vi "Save Waveform Chart history - single plot.vi"(8 "error in (no error)":errorcluster, 9 "History Data - singple plot":waveform(dbl)[](array[waveform]), 10 "Plot GUI label":string, 11 "Father of all uServices in":refnum<class "Father of all uServices.lvclass">) -> (0 "error out":errorcluster, 3 "Father of all uServices out":refnum<class "Father of all uServices.lvclass">)   [LabVIEW 2026, in "TALOS.lvlib" / "Father of all uServices.lvlib" / "Father of all uServices.lvclass"]
uses:
  Father of all uServices.lvclass
  Waveform Chart Class Reference Strict - single plot.ctl
  Ancestor/Ancestor/Ancestor.lvclass/Ancestor.ctl
  Support VIs/Generate Error.vi
  FGV/Error Memory/Get Error Description.vi
  Support VIs/Get PC name.vi
  Ancestor/Ancestor/Read ID.vi
  Support VIs/Get Class Name.vi
  <vilib>/Utility/error.llb/Clear Errors.vi
  FGV/Error Memory/Error Memory Core.vi
  <vilib>/AdvancedString/Delimited String to 1D String Array.vi
  <vilib>/AdvancedString/Delimited String to 1D String Array (string).vi
  Support VIs/Circus Root Path.vi
  FGV/Error Memory/Error Crt Lvl checker.vi
  FGV/Error Memory/Error Memory Core.vi/40c8088d-b597-4017-91af-faa98e00292e.vi
  FGV/Error Memory/Error Memory Core.vi/d4a3ab98-063c-4e44-b43d-fbdcfe6c2be2.vi
  <vilib>/Utility/file.llb/Write Delimited Spreadsheet (DBL).vi
  Support VIs/Global Memory.vi
  <vilib>/Utility/LVClass/Get LV Class Name.vi
  Support VIs/Is in Packed Library.vi
  Support VIs/TALOS Root path.vi
  Support VIs/Read CSV worksheet.vi
  Support VIs/Global Constants.vi
  <vilib>/Utility/error.llb/General Error Handler.vi
  Support VIs/Error Log.vi
  Ancestor/Ancestor/Ancestor.lvclass
  <vilib>/Comparison/Equal/Equal Functor/Equal Functor.lvclass
  TALOS.lvlib
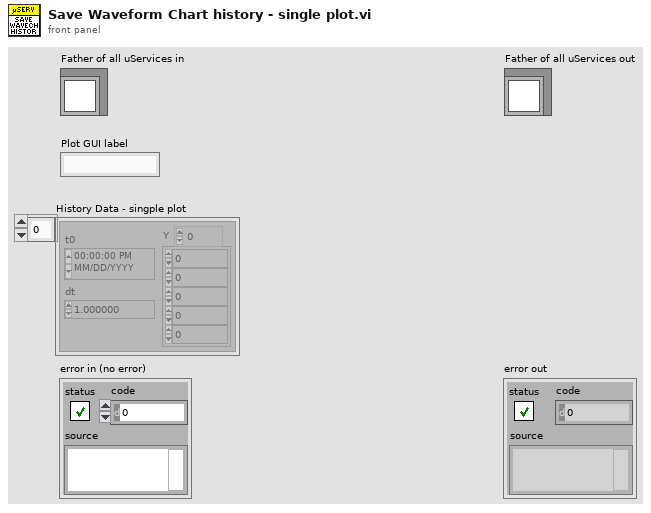
[diagram p1: front panel]
types:
  T1 = typedef "TALOS.lvlib/Father of all uServices.lvlib/Father of all uServices.lvclass/Waveform Chart Class Reference Strict - single plot.ctl" = refnum<vi>
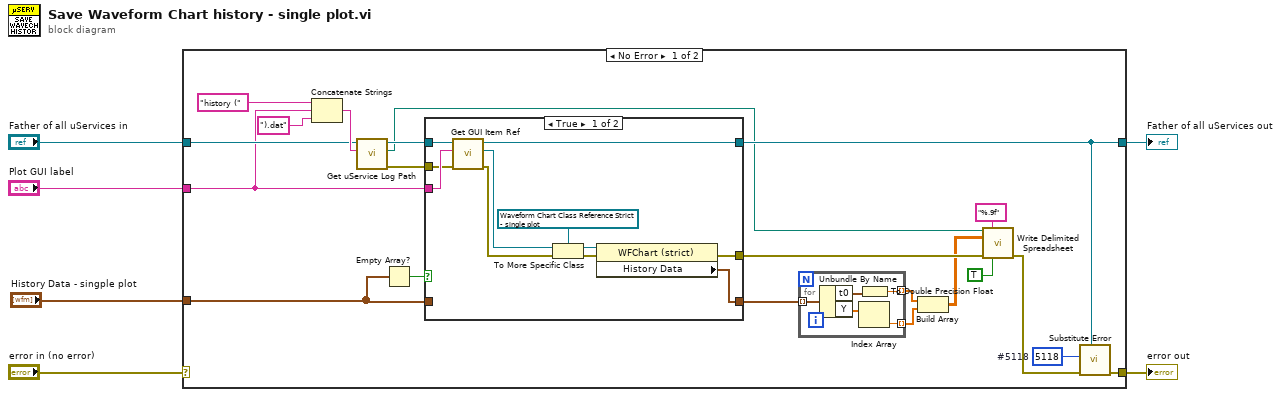
[diagram p0: block diagram]
diagram:
  n1 = case shown="No Error" "error in (no error)" {
    selector: "error in (no error)" -> [_ w48]
    tunnel: [w23 w48] -> w5
    tunnel: [w17 w47] -> w3
    tunnel: "Father of all uServices in" -> [w20 w47]
    tunnel: "Plot GUI label" -> [w16 _]
    tunnel: "History Data - singple plot" -> [w18 _]
    frame No Error {
      w22 = 5118  # #5118
      n2 = Concatenate Strings("history (" ("string"), w16, ").dat" ("string")) -> (w24:string)
      n3 = call "Get uService Log Path.vi"("Log File Suffix"=w24, "Father of all uServices in"=w20) -> ("error out"=w15:errorcluster, "Log File Path"=w13:path, "Father of all uServices out"=w19:refnum<class "Father of all uServices.lvclass">)  [unwired: 7 in]
      n4 = Empty Array?(array=w18) -> (empty?=w21:bool)
      n5 = case shown="True" w21 {
        tunnel: [w43 w44] -> w27
        tunnel: w19 -> [w40 w45]
        tunnel: w18 -> [_ w46]
        tunnel: [w39 w45] -> w17
        tunnel: w16 -> [w38 _]
        tunnel: [w36 w46] -> w14
        tunnel: w15 -> [w35 w44]
        frame True {
          n6 = call "Get GUI Item Ref.vi"("error in (no error)"=w35, "FP Item Name"=w38, "uService Template in"=w40) -> ("error out"=w34:errorcluster, "Ctl Refnum"=w37:refnum<vi>, "uService Template out"=w39:refnum<class "Father of all uServices.lvclass">)  [unwired: 6 in]
          n7 = To More Specific Class(target class=T1 refnum ("WFChart Refnum"), reference=w37, error in=w34) -> (specific class reference=w42:T1, error out=w41:errorcluster)
          n8 = property class="WFChart (strict)"(reference=w42, error in=w41) -> (error out=w43:errorcluster, "History Data"=w36:waveform(dbl)[])  [unwired: 1 out]
        }
        frame False {
        }
      }
      n9 = for {
        tunnel: w14 -> [w32] mode=indexing
        tunnel: [w29] -> w10 mode=indexing
        tunnel: [w28] -> w9 mode=indexing
        n10 = Unbundle By Name(w32) -> ("t0"=w30:timestamp, "Y"=w31:dbl[])
        n11 = Index Array(array=w31) -> (element=w28:dbl)  [unwired: 1 in]
        n12 = To Double Precision Float(number=w30) -> (double precision float=w29:dbl)
      }
      n13 = Build Array(w10, w9) -> (w8:dbl[][])
      n14 = call-poly <vilib>:"Write Delimited Spreadsheet.vi"("file path (dialog if empty)"=w13, "format (%.3f)"="%.9f", "2D data"=w8, "error in (no error)"=w27, "transpose? (no:F)"=TRUE) -> ("error out"=w12:errorcluster)  [unwired: 9 in, 1 out]
      n15 = call "Substitute Error.vi"("LabVIEW Object"=w17, "error in (no error)"=w12, "Error Code"=w22) -> ("error out"=w23:errorcluster)  [unwired: 8 in]
    }
    frame Error {
    }
  }
  "error out" <- w5
  "Father of all uServices out" <- w3
